vi "Panel.vi"(11 "SubClone in":refnum<class "SubClone.lvclass">) -> ()   [LabVIEW 2020, in "SubPanels.lvlib" / "SubClone.lvclass"]
uses:
  SubClone.lvclass
  C:/dev/lv-oopanel/OOPanel/Panel/Panel.lvclass
  SubClone.lvclass/SubClone.ctl
  OOPanel/Panel/Panel.lvclass
  OOPanel/OOPanel.lvlib
panel:
  out "Iterations":i32
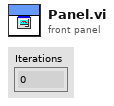
[diagram p1: front panel]
types:
  T1 = typedef "eventsource.ctl" = u32
  T2 = typedef "OOPanel.lvlib/Panel.lvclass/Visibility State.ctl" = enum16{"Idle", "Closed", "Hidden", "Visible", "Subpanel"}
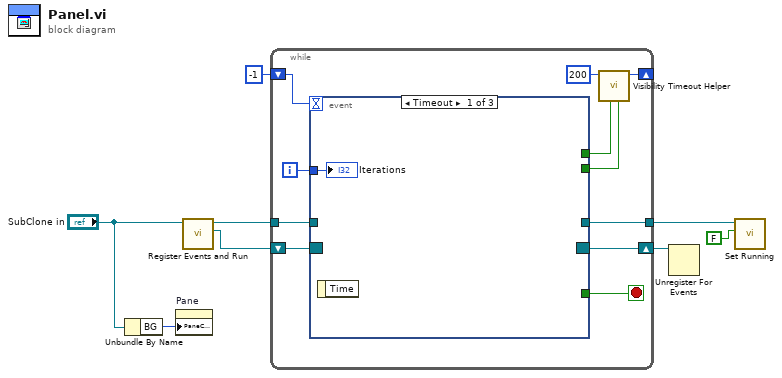
[diagram p0: block diagram]
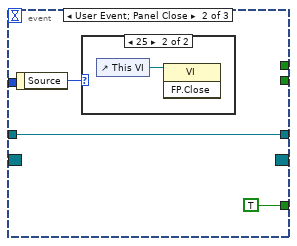
[diagram p2: hidden frame]
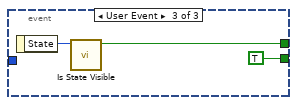
[diagram p4: hidden frame]
diagram:
  n1 = Unbundle By Name("SubClone in") -> ("BG"=w8:u32)
  n2 = property on="Pane" class="Pane"("PaneColor"=w8) -> ()  [unwired: 2 in, 2 out]
  n3 = call "Register Events and Run.vi"("Panel in"="SubClone in") -> ("Panel Event Reg"=w6:refnum<event-registration>, "Panel out"=w7:refnum<class "SubClone.lvclass">)  [unwired: 8 in, 1 out]
  n4 = while {
    tunnel: w7 -> [w10]
    shift-right: [w18] -> w2
    shift-left: w6 -> [w19]
    shift-right: [w16] -> _
    shift-left: -1 -> [w15]
    tunnel: [w9] -> w4
    i -> [w12]
    stop <- w11 stop-if-true
    n5 = event shown="[0] Timeout" {
      selector: w19 -> [_ _ _]
      dyn-events: [_ _ _] -> w18
      timeout: w15 -> [_ _ _]
      tunnel: [_ _ w26] -> w14
      tunnel: [_ _ TRUE] -> w13
      tunnel: w12 -> [w20 _ _]
      tunnel: [_ TRUE _] -> w11
      tunnel: w10 -> [_ w22 _]
      tunnel: [_ w22 _] -> w9
      event Timeout {
        n6 = event-data() -> ()  [unwired: 1 in, 1 out]
        "Iterations" <- w20
      }
      event User Event; Panel Close {
        n7 = event-data() -> ("Source"=w21:T1)  [unwired: 1 in]
        n8 = case shown="25" w21 {
          frame Default {
          }
          frame 25 {
            n9 = control-ref of="This VI"() -> (w24:refnum<vi>)
            n10 = invoke class="VI" method="FP.Close"(reference=w24) -> ()  [unwired: 2 in, 3 out]
          }
        }
      }
      event User Event {
        n11 = event-data() -> ("State"=w27:T2)  [unwired: 1 in]
        n12 = call "Is State Visible.vi"("Visibility"=w27) -> ("Visible"=w26:bool)  [unwired: 10 in]
      }
    }
    n13 = call "Visibility Timeout Helper.vi"("Update?"=w13, "Use Timeout?"=w14, "Visible Timeout mS"=200) -> ("Timeout"=w16:i32)  [unwired: 8 in]
  }
  n14 = Unregister For Events(event registration refnum=w2) -> ()  [unwired: 1 in, 1 out]
  n15 = call "Set Running.vi"("Running"=FALSE, "Panel in"=w4) -> ()  [unwired: 8 in, 2 out]
